vi "Master data typecast.vi"(2 "Data in":u8[](array[numeric])) -> (0 "Data out":T2, 1 "Datatype":T1(ring))   [LabVIEW 2016]
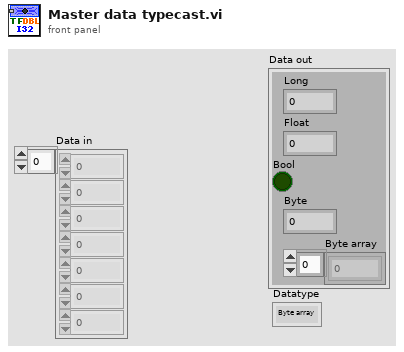
[diagram p1: front panel]
types:
  T1 = enum16{"Byte array", "Byte", "Bool", "Long", "Float"}
  T2 = cluster{"Long":i32, "Float":dbl, "Bool":bool, "Byte":u8, "Byte array":u8[]}
  T3 = enum16{"big-endian, network order", "native, host order", "little-endian"}
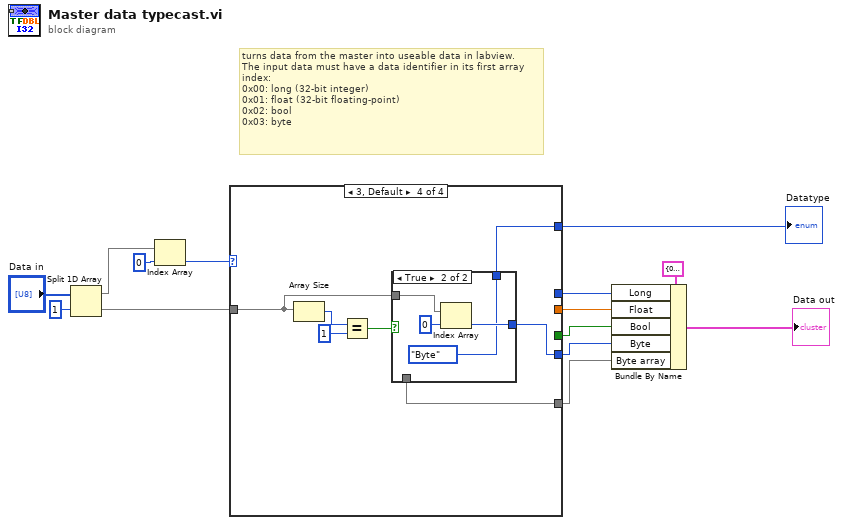
[diagram p0: block diagram]
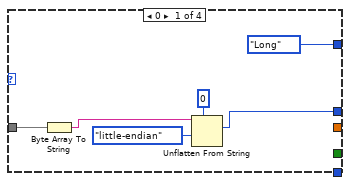
[diagram p2: hidden frame]
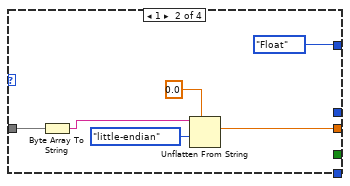
[diagram p3: hidden frame]
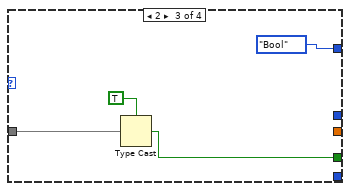
[diagram p4: hidden frame]
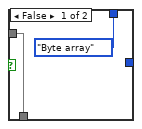
[diagram p5: hidden frame]
diagram:
  # "turns data from the master into useable data in labview.\nThe input data must have a data identifier in its first array\nindex:\n0x00: long (32-bit integer)\n0x01: float (32-bit floating-point)\n0x02: bool\n0x03: byte"
  n1 = Split 1D Array(array="Data in", index=1) -> (first subarray=w11:u8[], second subarray=w9:u8[])
  n2 = Index Array(array=w11, index=0) -> (element=w10:u8)
  n3 = case shown="3, Default" w10 {
    tunnel: w9 -> [w16 w23 w30 w35]
    tunnel: [w15 _ _ _] -> w7
    tunnel: [_ w24 _ _] -> w6
    tunnel: [_ _ w29 _] -> w5
    tunnel: [_ _ _ w34] -> w4
    tunnel: [_ _ _ w32] -> w3
    tunnel: [T1."Long" T1."Float" T1."Bool" w31] -> w1
    frame 0 {
      n4 = Byte Array To String(unsigned byte array=w16) -> (string=w18:string)
      n5 = Unflatten From String(type=0, binary string=w18, byte order (0:big-endian, network order)=T3."little-endian") -> (value=w15:i32)  [unwired: 2 in, 2 out]
    }
    frame 1 {
      n6 = Byte Array To String(unsigned byte array=w23) -> (string=w22:string)
      n7 = Unflatten From String(type=sgl 0.0, binary string=w22, byte order (0:big-endian, network order)=T3."little-endian") -> (value=w24:sgl)  [unwired: 2 in, 2 out]
    }
    frame 2 {
      n8 = Type Cast(type=TRUE, x=w30) -> (*(type *) &x=w29:bool)
    }
    frame 3, Default {
      n9 = Array Size(array=w35) -> (size(s)=w37:i32)
      n10 = Equal?(x=w37, y=1) -> (x = y?=w33:bool)
      n11 = case shown="True" w33 {
        tunnel: w35 -> [w39 w43]
        tunnel: [_ w41] -> w34
        tunnel: [w39 _] -> w32
        tunnel: [T1."Byte array" T1."Byte"] -> w31
        frame False {
        }
        frame True {
          n12 = Index Array(array=w43, index=0) -> (element=w41:u8)
        }
      }
    }
  }
  "Datatype" <- w1
  n13 = Bundle By Name(cluster=T2 {"Long"=0, "Float"=0.0, "Bool"=TRUE, "Byte"=0, "Byte array"=[]} ("input cluster"), "Long"=w7, "Float"=w6, "Bool"=w5, "Byte"=w4, "Byte array"=w3) -> (→"Data out":T2)
